vi "Main VI.vi"() -> ()   [LabVIEW 2020]
panel:
  out "Waveform Chart":dbl(graph)
  in  "Stop":bool
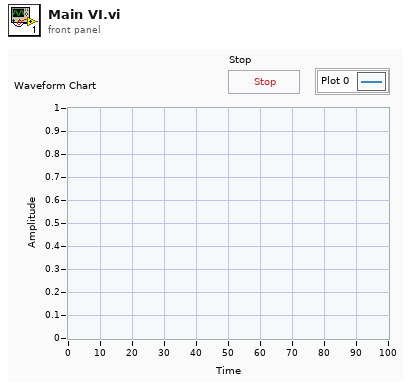
[diagram p1: front panel]
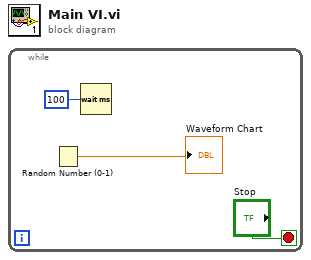
[diagram p0: block diagram]
diagram:
  n1 = while {
    stop <- "Stop" stop-if-true
    n2 = Random Number (0-1)() -> (number: 0 to 1=→"Waveform Chart":dbl)
    n3 = Wait (ms)(milliseconds to wait=u32 100) -> ()  [unwired: 1 out]
  }
